vi "Main.vi"() -> ()   [LabVIEW 2023]
uses:
  SubVIs/Functions.lvlib
panel:
  out "Result":dbl
  in  "Divide":bool
  in  "Multiply":bool
  in  "Subtract":bool
  in  "Add":bool
  in  "Operand 2":dbl
  in  "Operand 1":dbl
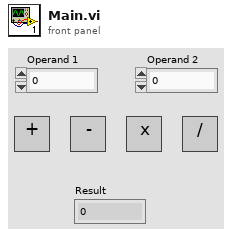
[diagram p1: front panel]
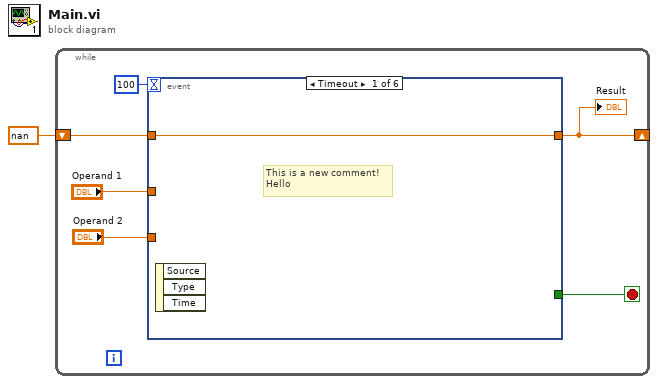
[diagram p0: block diagram]
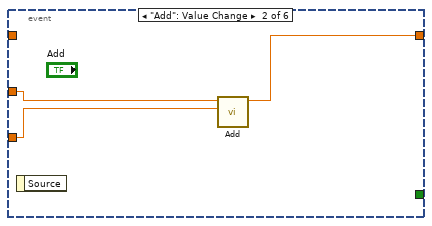
[diagram p2: hidden frame]
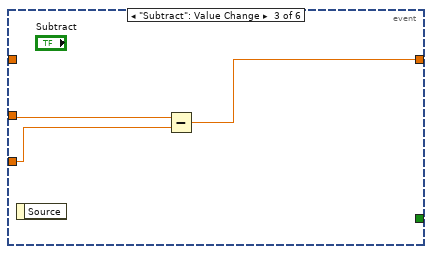
[diagram p3: hidden frame]
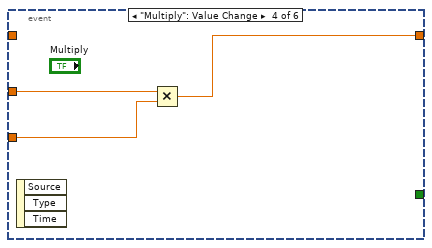
[diagram p4: hidden frame]
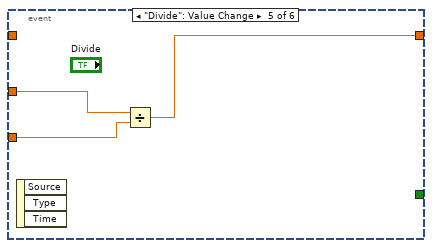
[diagram p5: hidden frame]
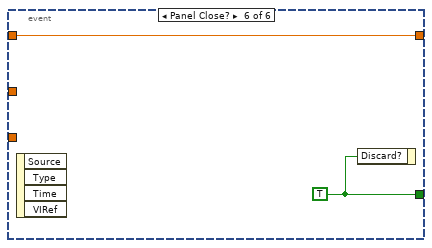
[diagram p6: hidden frame]
diagram:
  n1 = while {
    shift-right: [w2] -> _
    shift-left: nan ("Numeric") -> [w3]
    stop <- w4 stop-if-true
    n2 = event shown="[0] Timeout" {
      selector: _ -> [_ _ _ _ _ _]
      dyn-events: _ -> [_ _ _ _ _ _]
      timeout: 100 -> [_ _ _ _ _ _]
      tunnel: "Operand 1" -> [_ w11 w14 w17 w20 _]
      tunnel: "Operand 2" -> [_ w10 w13 w16 w19 _]
      tunnel: [_ _ _ _ _ w22] -> w4
      tunnel: w3 -> [w8 _ _ _ _ w21]
      tunnel: [w8 w9 w12 w15 w18 w21] -> w2
      event Timeout {
        # "This is a new comment!\nHello"
        n3 = event-data() -> ()  [unwired: 1 in, 3 out]
      }
      event "Add": Value Change {
        n4 = event-data() -> ()  [unwired: 1 in, 1 out]
        n5 = call "Add.vi"("Operand 2"=w10, "Operand 1"=w11) -> ("Numeric"=w9:dbl)  [unwired: 9 in]
      }
      event "Subtract": Value Change {
        n6 = event-data() -> ()  [unwired: 1 in, 1 out]
        n7 = Subtract(x=w14, y=w13) -> (x-y=w12:dbl)
      }
      event "Multiply": Value Change {
        n8 = event-data() -> ()  [unwired: 1 in, 3 out]
        n9 = Multiply(x=w17, y=w16) -> (x*y=w15:dbl)
      }
      event "Divide": Value Change {
        n10 = event-data() -> ()  [unwired: 1 in, 3 out]
        n11 = Divide(x=w20, y=w19) -> (x/y=w18:dbl)
      }
      event Panel Close? {
        w22 = TRUE
        n12 = event-data() -> ()  [unwired: 1 in, 4 out]
        n13 = event-data("Discard?"=w22) -> ()  [unwired: 1 in, 1 out]
      }
    }
    "Result" <- w2
  }
